vi "CanOpen Interface.vi"(8 "error in (no error)":errorcluster caption="Fehler (Eingang, kein Fehler)", 11 "S706 CanOpen Eingang":refnum<class "S706 CanOpen.lvclass"> caption="DNL_LabVIEW Object in") -> (0 "error out":errorcluster caption="Fehler (Ausgang)", 3 "S706 CanOpen Ausgang":refnum<class "S706 CanOpen.lvclass"> caption="DNL_LabVIEW Object out")   [LabVIEW 2013, in "S706 CanOpen.lvclass"]
uses:
  S706 CanOpen.lvclass
  S706 CanOpen.lvclass/S706 CanOpen.ctl
  <vilib>/CANopenLib/CANOPEN.llb/CANopen Interface Create.vi
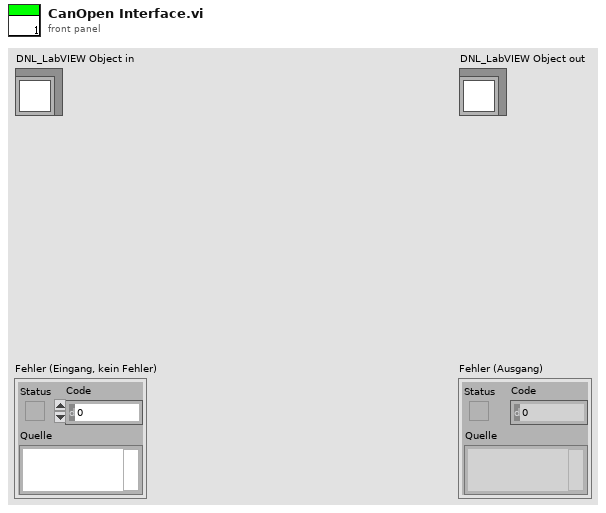
[diagram p1: front panel]
types:
  T1 = typedef "CANopen BaudRate.ctl" = u32
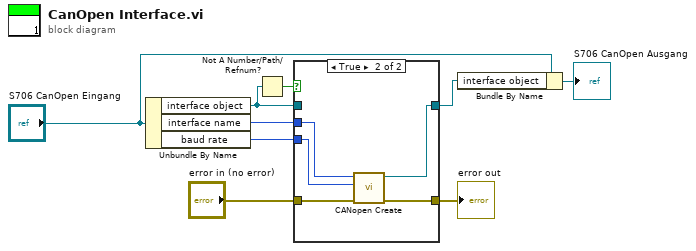
[diagram p0: block diagram]
diagram:
  n1 = Unbundle By Name("S706 CanOpen Eingang") -> ("interface object"=w1:refnum<k20>, "interface name"=w3:u32, "baud rate"=w2:T1)
  n2 = Not A Number/Path/Refnum?(number/path/refnum=w1) -> (NaN/Path/Refnum?=w5:bool)
  n3 = case shown="True" w5 {
    tunnel: "error in (no error)" -> [w11 w16]
    tunnel: [w11 w15] -> w8
    tunnel: [w10 w14] -> w4
    tunnel: w3 -> [_ w12]
    tunnel: w2 -> [_ w13]
    tunnel: w1 -> [w10 _]
    frame False {
    }
    frame True {
      n4 = call-poly <vilib>:"CANopen Create.vi"("error in (no error)"=w16, "baud rate"=w13, "interface name"=w12) -> ("error out"=w15:errorcluster, "interface object out"=w14:refnum<k20>)  [unwired: 7 in]
    }
  }
  "error out" <- w8
  n5 = Bundle By Name(cluster="S706 CanOpen Eingang", "interface object"=w4) -> (→"S706 CanOpen Ausgang":refnum<class "S706 CanOpen.lvclass">)
